vi "dfd_CIC_Interpolation.vi"(0 "input data":fxp<+/-,32,32>, 9 "input valid":bool) -> (4 "output data":fxp<+/-,32,32>=-256.0, 10 "output valid":bool=TRUE, 14 "ready for input":bool=TRUE)   [LabVIEW 2017]
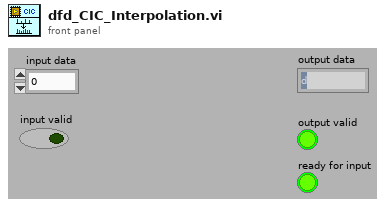
[diagram p1: front panel]
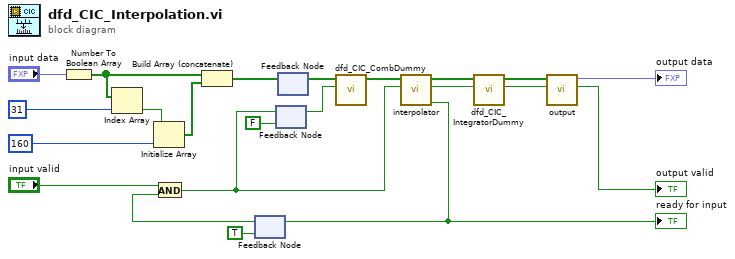
[diagram p0: block diagram]
diagram:
  n1 = Number To Boolean Array(number="input data") -> (Boolean array=w18:bool[])
  n2 = Index Array(array=w18, index=31 ("input msb")) -> (element=w19:bool)
  n3 = Initialize Array(w19, 160 ("192-input wl")) -> (w21:bool[])
  n4 = Build Array (concatenate)(w18, w21) -> (w16:bool[])
  n5 = feedback #1(TRUE ("ready for input")) -> (w2:bool)
  n6 = And(x="input valid", y=w2) -> (x .and. y?=w1:bool)
  n7 = feedback-in #2(w1) -> ()
  n8 = feedback #2(FALSE ("input valid")) -> (w5:bool)
  n9 = feedback-in #3(w16) -> ()
  n10 = feedback #3() -> (w6:bool[])  [unwired: 1 out]
  n11 = call <vilib>:"dfd_CIC_CombDummy.vi"("input valid"=w5, "data in"=w6) -> ("data out"=w11:bool[])  [unwired: 9 out]
  n12 = call "interpolator"("input valid"=w1, "input data"=w11) -> ("ready for input"=w14:bool, "output valid"=w9:bool, "output data"=w10:bool[])  [unwired: 7 out]
  "ready for input" <- w14
  n13 = feedback-in #1(w14) -> ()
  n14 = call <vilib>:"dfd_CIC_IntegratorDummy.vi"("input valid"=w9, "data in"=w10) -> ("output valid"=w7:bool, "data out"=w8:bool[])  [unwired: 8 out]
  n15 = call "output"("input valid"=w7, "input data"=w8) -> ("output valid"=→"output valid":bool, "output data"=→"output data":fxp<+/-,32,32>)  [unwired: 8 in]
